vi "MP-285 Reach Position.vi"(2 "cluster":errorcluster, 3 "Output: VISA session OUT":refnum<visa-resource-name>) -> (0 "cluster 2":errorcluster, 1 "Output: VISA session OUT 2":refnum<visa-resource-name>)   [LabVIEW 2010]
uses:
  StageMG100204SutterMP285/StageMG100204SutterMP285.lvclass
panel:
  out "Boolean":bool
  # "Waiting for the manipulator"
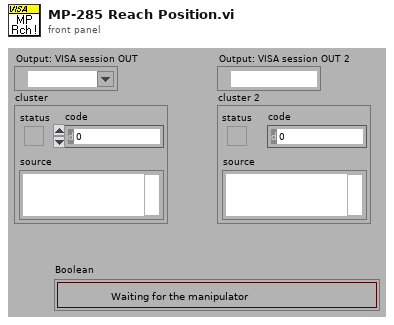
[diagram p1: front panel]
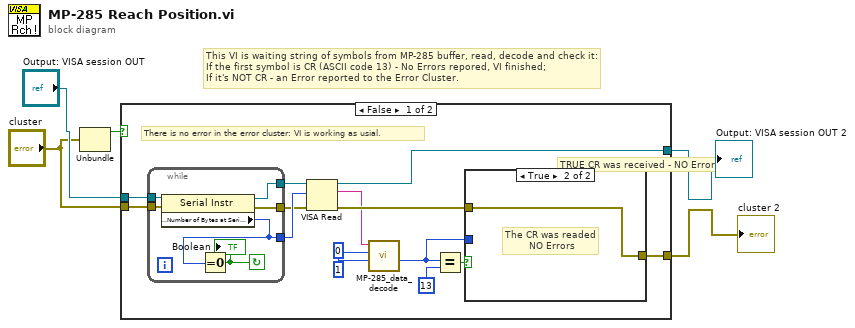
[diagram p0: block diagram]
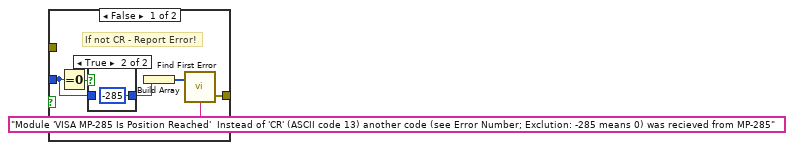
[diagram p2: hidden frame]
diagram:
  # "This VI is waiting string of symbols from MP-285 buffer, read, decode and check it:\nIf the first symbol is CR (ASCII code 13) - No Errors repored, VI finished;\nIf it's NOT CR - an Error reported to the Error Cluster."
  n1 = Unbundle("cluster") -> ("status"=w5:bool)  [unwired: 2 out]
  n2 = case shown="False" w5 {
    tunnel: "cluster" -> [w16 w35]
    tunnel: "Output: VISA session OUT" -> [w15 w36]
    tunnel: [w11 w35] -> w3
    tunnel: [w9 w36] -> w4
    frame False {
      # "There is no error in the error cluster: VI is working as usial."
      n3 = while {
        tunnel: w16 -> [w34]
        tunnel: [w33] -> w17
        tunnel: w15 -> [w32]
        tunnel: [w31] -> w18
        tunnel: [w30] -> w19
        stop <- w29 continue-if-true
        n4 = property class="Serial Instr"(reference=w32, error in=w34) -> (reference out=w31:refnum<visa-resource-name>, error out=w33:errorcluster, "Serial Settings:Number of Bytes at Serial Port"=w30:u32)
        n5 = Equal To 0?(x=w30) -> (x = 0?=w29:bool)
        "Boolean" <- w29
      }
      n6 = VISA Read(VISA resource name=w18, byte count=w19, error in (no error)=w17) -> (VISA resource name out=w9:refnum<visa-resource-name>, read buffer=w8:string, error out=w10:errorcluster)  [unwired: 1 out]
      n7 = call "MP-285_data_decode.vi"("length"=0, "offset"=1, "encoded data string in"=w8) -> ("decoded data"=w12:i32)  [unwired: 6 in, 2 out]
      n8 = Equal?(x=w12, y=13) -> (x = y?=w14:bool)
      n9 = case shown="True" w14 {
        tunnel: [w25 w28] -> w11
        tunnel: w12 -> [w20 _]
        tunnel: w10 -> [_ w28]
        frame False {
          # "If not CR - Report Error!"
          n10 = Equal To 0?(x=w20) -> (x = 0?=w22:bool)
          n11 = case shown="True" w22 {
            tunnel: [w26 -285] -> w21
            tunnel: w20 -> [w26 _]
            frame False {
            }
            frame True {
            }
          }
          n12 = Build Array(w21) -> (w24:i32[])
          n13 = call <vilib>:"Find First Error.vi"("source messages"="Module 'VISA MP-285 Is Position Reached'  Instead of 'CR' (ASCII code 13) another code (see Error Number; Exclution: -285 means 0) was recieved from MP-285", "error codes"=w24) -> ("error out"=w25:errorcluster)  [unwired: 1 in, 2 out]
        }
        frame True {
          # "The CR was readed\n        NO Errors"
          # "TRUE CR was received - NO Errors"
        }
      }
    }
    frame True {
      # "There is an Error in Error Cluster - this VI should do nothing."
    }
  }
  "Output: VISA session OUT 2" <- w4
  "cluster 2" <- w3
